vi "Begin.vi"() -> (0 "error out":errorcluster)   [LabVIEW 2012]
doc: "Called before other user functions, this VI is expected to open initial I/O refnums, load in file data, and do all program initialization. Notice that the <B>error out</B> terminal is simply used for data flow. Wiring it to other structures or subVIs ensures that this VI runs first."
uses:
  <vilib>/Rock Robotics/WPI/Joystick/WPI_JoystickDeviceEnum.ctl
  <vilib>/Rock Robotics/SystemInterfaces/Typedef/FPGA_TypedefDigitalModule.ctl
  <vilib>/Rock Robotics/SystemInterfaces/Typedef/FPGA_TypedefSolenoidModule.ctl
  <vilib>/Rock Robotics/WPI/Solenoid/WPI_SolenoidChannel.ctl
  <vilib>/Rock Robotics/WPI/Solenoid/WPI_SolenoidValue.ctl
  <vilib>/Rock Robotics/WPI/Camera/WPI_CameraImageSize.ctl
  <vilib>/Rock Robotics/WPI/Camera/WPI_CameraWhite Balance Values.ctl
  <vilib>/Rock Robotics/WPI/Camera/WPI_CameraExposure Values.ctl
  <vilib>/Rock Robotics/WPI/Camera/WPI_CameraFrameRate.ctl
  <vilib>/Rock Robotics/SystemInterfaces/DIO/FPGA_DIOChannel.ctl
  <vilib>/Rock Robotics/SystemInterfaces/DIO/FPGA_DIORelayChannel.ctl
  <vilib>/Rock Robotics/SystemInterfaces/DIO/FPGA_DIOPWMChannel.ctl
  <vilib>/Rock Robotics/WPI/Solenoid/WPI_SolenoidOpenDouble.vi
  <vilib>/Rock Robotics/WPI/Solenoid/WPI_SolenoidSetEnum.vi
  <vilib>/Rock Robotics/WPI/Compressor/WPI_CompressorGetSetRefNum.vi
  <vilib>/Rock Robotics/WPI/Counter/WPI_CounterDigitalInputToDigitalSource.vi
  <vilib>/Rock Robotics/WPI/MotorControl/WPI_MotorControlOpen Victor.vi
  <vilib>/Rock Robotics/WPI/RobotDrive/WPI_RobotDriveOpen2MotorWithVictor.vi
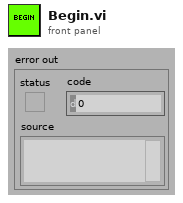
[diagram p1: front panel]
types:
  T1 = typedef "WPI_JoystickDeviceEnum.ctl" = enum16{"USB 1", "USB 2", "USB 3", "USB 4", "Kinect 1", "Kinect 2"}
  T2 = typedef "FPGA_TypedefDigitalModule.ctl" = enum16{"Digital Module 1", "Digital Module 2"}
  T3 = typedef "WPI_CameraFrameRate.ctl" = u32
  T4 = typedef "WPI_CameraExposure Values.ctl" = enum16{"Auto", "Flicker-free 50 Hz", "Flicker-free 60 Hz", "Hold current"}
  T5 = typedef "WPI_CameraWhite Balance Values.ctl" = enum16{"Auto", "Fixed indoor", "Fixed outdoor 1", "Fixed outdoor 2", "Fixed fluorescent 1", "Fixed fluorescent 2", "Hold current"}
  T6 = typedef "WPI_CameraImageSize.ctl" = enum16{"640x480", "320x240", "160x120"}
  T7 = typedef "WPI_CameraDevRef.ctl" = cluster{"Camera Address":string, "CameraStatus":errorcluster, "Acquire Image Notifier":refnum<notifier>}
  T8 = typedef "FPGA_DIOChannel.ctl" = enum8{"DIO 1", "DIO 2", "DIO 3", "DIO 4", "DIO 5", "DIO 6", "DIO 7", "DIO 8", "DIO 9", "DIO 10", "DIO 11", "DIO 12", "DIO 13", "DIO 14", "Invalid"}
  T9 = typedef "FPGA_DIOPWMChannel.ctl" = enum8{"PWM 1", "PWM 2", "PWM 3", "PWM 4", "PWM 5", "PWM 6", "PWM 7", "PWM 8", "PWM 9", "PWM 10", "Invalid"}
  T10 = typedef "WPI_DigitalInputDevRef.ctl" = cluster{"DevStatus":errorcluster, "DIO Channel":T8, "Digital Module":T2}
  T11 = typedef "WPI_RobotDriveDevRef.ctl" = cluster{"DevStatus":errorcluster, "Motors[]":T12[], "Square Inputs":bool, "Max Output":dbl, "Isochronous":bool}
  T12 = typedef "WPI_MotorControlDeviceRef.ctl" = cluster{"DeviceStatus":errorcluster, "Type":enum16{"PWM", "CAN"}, "PWM":cluster{"Digital Module":T2, "PWM Channel":T9, "DeadBand":T13}, "CAN":cluster{"Device Number":u8, "Control Mode":T14, "Semaphore":T15, "Max Vout":dbl}, "Invert":bool, "TransformRef":T16, "InvTransformRef":T16}
  T13 = typedef "WPI_PWMDeadband.ctl" = cluster{"Name":string, "maxPositivePwm":i32, "minPositivePwm":i32, "centerPwm":i32, "maxNegativePwm":i32, "minNegativePwm":i32, "angularRange":u16}
  T14 = typedef "WPI_CANJaguar_ControlMode.ctl" = enum8{"Percent VBus", "Current", "Speed", "Position", "Voltage"}
  T15 = typedef "Semaphore RefNum" = refnum<k1>
  T16 = typedef "WPI_PWMTransform_ConPane.ctl" = refnum<vi>
  T17 = typedef "FPGA_CounterEncoderSourceConvertionLVSourceType.ctl" = cluster{"DevStatus":errorcluster, "AnalogTriggerMode?":bool, "DigitalMode":cluster{"Digital Module":T2, "DIO Channel":T18}, "AnalogTriggerMode":cluster{"AnalogTriggerIndex":T19, "OutputType":T20}}
  T18 = typedef "FPGA_DIODigitalSourceChannel.ctl" = enum8{"DIO 1", "DIO 2", "DIO 3", "DIO 4", "DIO 5", "DIO 6", "DIO 7", "DIO 8", "DIO 9", "DIO 10", "DIO 11", "DIO 12", "DIO 13", "DIO 14", "Disabled"}
  T19 = typedef "FPGA_AnalogTriggerIndex.ctl" = enum8{"Trig 0", "Trig 1", "Trig 2", "Trig 3", "Trig 4", "Trig 5", "Trig 6", "Trig 7", "Invalid"}
  T20 = typedef "FPGA_AnalogTriggerOutType.ctl" = enum16{"InWindow", "TriggerState", "Rising", "Falling"}
  T21 = typedef "WPI_EncoderDevRef.ctl" = cluster{"DevStatus":errorcluster, "EncoderIndex":T22, "CounterIndex":T23, "DistancePerCount":dbl, "Decoding Type":T24}
  T22 = typedef "FPGA_EncoderIdx.ctl" = enum8{"Enc 0", "Enc 1", "Enc 2", "Enc 3", "Invalid"}
  T23 = typedef "FPGA_CounterCtrSystemIndex.ctl" = enum8{"Ctr 0", "Ctr 1", "Ctr 2", "Ctr 3", "Ctr 4", "Ctr 5", "Ctr 6", "Ctr 7", "Invalid"}
  T24 = typedef "WPI_EncoderType.ctl" = enum16{"1x", "2x", "4x"}
  T25 = typedef "WPI_SolenoidValue.ctl" = enum16{"Off", "On", "Forward", "Reverse"}
  T26 = typedef "WPI_SolenoidChannel.ctl" = enum8{"Solenoid 1", "Solenoid 2", "Solenoid 3", "Solenoid 4", "Solenoid 5", "Solenoid 6", "Solenoid 7", "Solenoid 8", "Invalid"}
  T27 = typedef "FPGA_TypedefSolenoidModule.ctl" = enum16{"Solenoid Module 1", "Solenoid Module 2"}
  T28 = typedef "WPI_SolenoidDevRef.ctl" = cluster{"DevStatus":errorcluster, "Solenoid Module":T27, "Forward Solenoid Channel":T26, "Reverse Solenoid Channel":T26}
  T29 = typedef "FPGA_DIORelayChannel.ctl" = enum8{"Relay 1", "Relay 2", "Relay 3", "Relay 4", "Relay 5", "Relay 6", "Relay 7", "Relay 8", "Invalid"}
  T30 = typedef "WPI_CompressorDevRef.ctl" = cluster{"DevStatus":errorcluster, "DigitalInputDevRef":T10, "RelayDevRef":T31}
  T31 = typedef "WPI_RelayDevRef.ctl" = cluster{"DevStatus":errorcluster, "Relay Channel":T29, "Digital Module":T2, "Relay Direction":T32}
  T32 = typedef "WPI_RelayDirection.ctl" = enum16{"Both directions", "Forward only", "Reverse only"}
  T33 = typedef "WPI_JoystickDevRef.ctl" = cluster{"Device":T1}
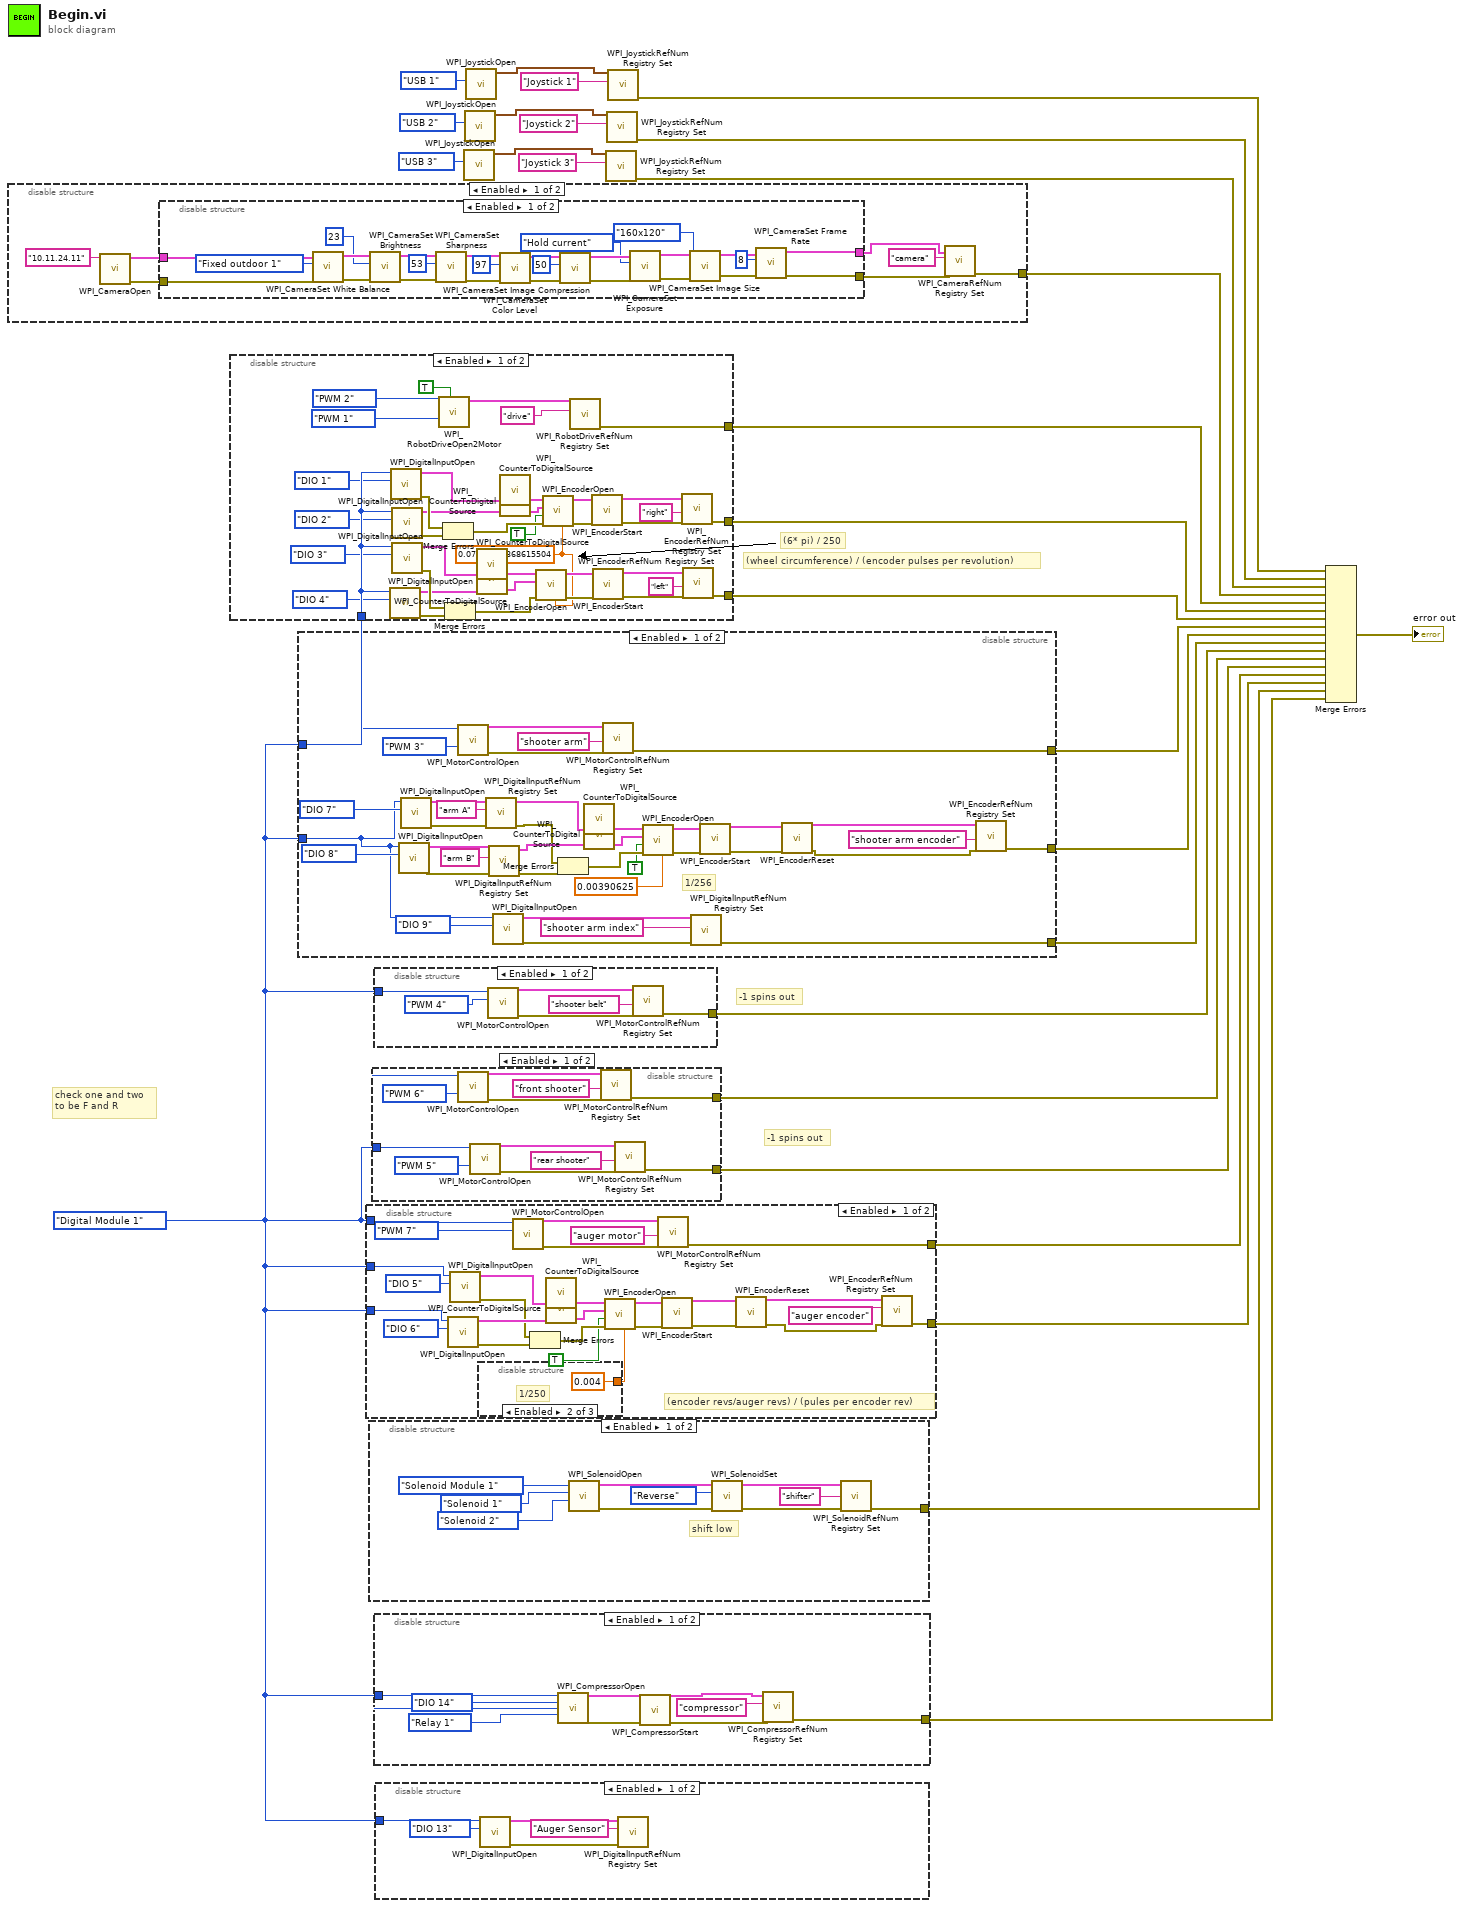
[diagram p0: block diagram]
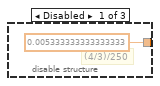
[diagram p4: hidden frame]
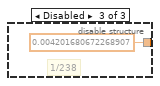
[diagram p5: hidden frame]
diagram:
  w1 = FPGA_TypedefDigitalModule."Digital Module 1" ("Digital Module (Module 1)")
  # "-1 spins out"
  # "-1 spins out"
  # "(wheel circumference) / (encoder pulses per revolution)"
  # "(6* pi) / 250"
  # "check one and two\nto be F and R"
  n1 = disable-structure shown="Enabled" {
    disable-tunnel: [w29 _] -> w16
    frame Enabled {
      n2 = call <vilib>:"WPI_CameraOpen.vi"("Camera Address"="10.11.24.11") -> ("error out"=w31:errorcluster, "CameraDevRef"=w33:T7)  [unwired: 9 in]
      n3 = disable-structure shown="Enabled" {
        disable-tunnel: w33 -> [w59 w63]
        disable-tunnel: [w37 w63] -> w32
        disable-tunnel: w31 -> [w46 w62]
        disable-tunnel: [w36 w62] -> w30
        frame Enabled {
          n4 = call <vilib>:"WPI_CameraSet White Balance.vi"("error in (no error)"=w46, "White Balance"=WPI_CameraWhite_Balance_Values."Fixed outdoor 1", "CameraDevRef"=w59) -> ("error out"=w47:errorcluster, "CameraDevRef Out"=w58:T7)  [unwired: 7 in]
          n5 = call <vilib>:"WPI_CameraSet Brightness.vi"("error in (no error)"=w47, "Brightness"=23, "CameraDevRef"=w58) -> ("error out"=w48:errorcluster, "CameraDevRef Out"=w57:T7)  [unwired: 7 in]
          n6 = call <vilib>:"WPI_CameraSet Sharpness.vi"("error in (no error)"=w48, "Sharpness"=53, "CameraDevRef"=w57) -> ("error out"=w49:errorcluster, "CameraDevRef Out"=w56:T7)  [unwired: 7 in]
          n7 = call <vilib>:"WPI_CameraSet Color Level.vi"("error in (no error)"=w49, "Color Level"=97, "CameraDevRef"=w56) -> ("error out"=w50:errorcluster, "CameraDevRef Out"=w55:T7)  [unwired: 7 in]
          n8 = call <vilib>:"WPI_CameraSet Image Compression.vi"("error in (no error)"=w50, "Compression"=50, "CameraDevRef"=w55) -> ("error out"=w61:errorcluster, "CameraDevRef Out"=w60:T7)  [unwired: 7 in]
          n9 = call <vilib>:"WPI_CameraSet Exposure.vi"("error in (no error)"=w61, "Exposure"=WPI_CameraExposure_Values."Hold current", "CameraDevRef"=w60) -> ("error out"=w51:errorcluster, "CameraDevRef Out"=w54:T7)  [unwired: 7 in]
          n10 = call <vilib>:"WPI_CameraSet Image Size.vi"("error in (no error)"=w51, "Image Size"=WPI_CameraImageSize."160x120", "CameraDevRef"=w54) -> ("error out"=w52:errorcluster, "CameraDevRef Out"=w53:T7)  [unwired: 7 in]
          n11 = call <vilib>:"WPI_CameraSet Frame Rate.vi"("error in (no error)"=w52, "Frame Rate (fps)"=T3 8, "CameraDevRef"=w53) -> ("error out"=w36:errorcluster, "CameraDevRef Out"=w37:T7)  [unwired: 7 in]
        }
        frame Disabled {
        }
      }
      n12 = call <vilib>:"WPI_CameraRefNum Registry Set.vi"("error in (no error)"=w30, "refnum name"="camera", "CameraDevRef"=w32) -> ("error out"=w29:errorcluster)  [unwired: 7 in, 1 out]
    }
    frame Disabled {
    }
  }
  n13 = disable-structure shown="Enabled" {
    disable-tunnel: w1 -> [w82 _]
    disable-tunnel: [w76 _] -> w15
    disable-tunnel: [w75 _] -> w14
    disable-tunnel: [w74 _] -> w13
    frame Enabled {
      w77 = 0.07539822368615504 ("DistancePerCount")
      n14 = call <vilib>:"WPI_DigitalInputOpen.vi"("DIO Channel"=FPGA_DIOChannel."DIO 4", "Digital Module (Module 1)"=w82) -> ("error out"=w73:errorcluster, "DigitalInputDevRef"=w66:T10)  [unwired: 8 in]
      n15 = call <vilib>:"WPI_DigitalInputOpen.vi"("DIO Channel"=FPGA_DIOChannel."DIO 1", "Digital Module (Module 1)"=w82) -> ("error out"=w68:errorcluster, "DigitalInputDevRef"=w86:T10)  [unwired: 8 in]
      n16 = call <vilib>:"WPI_DigitalInputOpen.vi"("DIO Channel"=FPGA_DIOChannel."DIO 2", "Digital Module (Module 1)"=w82) -> ("error out"=w70:errorcluster, "DigitalInputDevRef"=w67:T10)  [unwired: 8 in]
      n17 = call <vilib>:"WPI_DigitalInputOpen.vi"("DIO Channel"=FPGA_DIOChannel."DIO 3", "Digital Module (Module 1)"=w82) -> ("error out"=w71:errorcluster, "DigitalInputDevRef"=w100:T10)  [unwired: 8 in]
      n18 = call-poly <vilib>:"WPI_RobotDriveOpen2Motor.vi"("Left Motor Inverted"=TRUE, "Right Motor"=FPGA_DIOPWMChannel."PWM 1", "Left Motor"=FPGA_DIOPWMChannel."PWM 2") -> ("RobotDriveDevRef"=w102:T11)  [unwired: 7 in, 1 out]
      n19 = Merge Errors(w68, w70) -> (w69:errorcluster)
      n20 = Merge Errors(w71, w73) -> (w72:errorcluster)
      n21 = call-poly <vilib>:"WPI_CounterToDigitalSource.vi"("DigitalInputDevRef"=w100) -> ("Digital Source"=w93:T17)  [unwired: 6 in]
      n22 = call-poly <vilib>:"WPI_CounterToDigitalSource.vi"("DigitalInputDevRef"=w66) -> ("Digital Source"=w94:T17)  [unwired: 6 in]
      n23 = call-poly <vilib>:"WPI_CounterToDigitalSource.vi"("DigitalInputDevRef"=w86) -> ("Digital Source"=w92:T17)  [unwired: 6 in]
      n24 = call-poly <vilib>:"WPI_CounterToDigitalSource.vi"("DigitalInputDevRef"=w67) -> ("Digital Source"=w91:T17)  [unwired: 6 in]
      n25 = call <vilib>:"WPI_EncoderOpen.vi"("DistancePerCount"=w77, "error in (no error)"=w72, "BSource"=w94, "ASource"=w93) -> ("error out"=w95:errorcluster, "EncoderDevRef"=w96:T21)  [unwired: 6 in]
      n26 = call <vilib>:"WPI_EncoderOpen.vi"("DistancePerCount"=w77, "error in (no error)"=w69, "Invert Direction (False)"=TRUE, "BSource"=w91, "ASource"=w92) -> ("error out"=w90:errorcluster, "EncoderDevRef"=w89:T21)  [unwired: 5 in]
      n27 = call <vilib>:"WPI_RobotDriveRefNum Registry Set.vi"("refnum name"="drive", "RobotDriveDevRef"=w102) -> ("error out"=w76:errorcluster)  [unwired: 8 in, 1 out]
      n28 = call <vilib>:"WPI_EncoderStart.vi"("error in (no error)"=w90, "EncoderDevRef"=w89) -> ("error out"=w88:errorcluster, "EncoderDevRef"=w87:T21)  [unwired: 8 in]
      n29 = call <vilib>:"WPI_EncoderStart.vi"("error in (no error)"=w95, "EncoderDevRef"=w96) -> ("error out"=w97:errorcluster, "EncoderDevRef"=w98:T21)  [unwired: 8 in]
      n30 = call <vilib>:"WPI_EncoderRefNum Registry Set.vi"("error in (no error)"=w88, "refnum name"="right", "EncoderDevRef"=w87) -> ("error out"=w75:errorcluster)  [unwired: 7 in, 1 out]
      n31 = call <vilib>:"WPI_EncoderRefNum Registry Set.vi"("error in (no error)"=w97, "refnum name"="left", "EncoderDevRef"=w98) -> ("error out"=w74:errorcluster)  [unwired: 7 in, 1 out]
    }
    frame Disabled {
    }
  }
  n32 = disable-structure shown="Enabled" {
    disable-tunnel: w1 -> [w135 _]
    disable-tunnel: w1 -> [w125 _]
    disable-tunnel: [w121 _] -> w12
    disable-tunnel: [w120 _] -> w11
    disable-tunnel: [w119 _] -> w10
    frame Enabled {
      # "1/256"
      n33 = call <vilib>:"WPI_DigitalInputOpen.vi"("DIO Channel"=FPGA_DIOChannel."DIO 8", "Digital Module (Module 1)"=w125) -> ("error out"=w108:errorcluster, "DigitalInputDevRef"=w109:T10)  [unwired: 8 in]
      n34 = call <vilib>:"WPI_DigitalInputOpen.vi"("DIO Channel"=FPGA_DIOChannel."DIO 7", "Digital Module (Module 1)"=w125) -> ("error out"=w111:errorcluster, "DigitalInputDevRef"=w112:T10)  [unwired: 8 in]
      n35 = call-poly <vilib>:"WPI_MotorControlOpen.vi"("PWM Channel"=FPGA_DIOPWMChannel."PWM 3", "Digital Module (Module 1)"=w135) -> ("error out"=w137:errorcluster, "MotorControlDeviceRef"=w138:T12)  [unwired: 8 in]
      n36 = call <vilib>:"WPI_DigitalInputRefNum Registry Set.vi"("error in (no error)"=w111, "refnum name"="arm A", "DigitalInputDevRef"=w112) -> ("error out"=w104:errorcluster, "DigitalInputDevRef"=w106:T10)  [unwired: 7 in]
      n37 = call <vilib>:"WPI_DigitalInputRefNum Registry Set.vi"("error in (no error)"=w108, "refnum name"="arm B", "DigitalInputDevRef"=w109) -> ("error out"=w103:errorcluster, "DigitalInputDevRef"=w105:T10)  [unwired: 7 in]
      n38 = call <vilib>:"WPI_DigitalInputOpen.vi"("DIO Channel"=FPGA_DIOChannel."DIO 9", "Digital Module (Module 1)"=w125) -> ("error out"=w123:errorcluster, "DigitalInputDevRef"=w124:T10)  [unwired: 8 in]
      n39 = Merge Errors(w104, w103) -> (w118:errorcluster)
      n40 = call-poly <vilib>:"WPI_CounterToDigitalSource.vi"("DigitalInputDevRef"=w106) -> ("Digital Source"=w133:T17)  [unwired: 6 in]
      n41 = call-poly <vilib>:"WPI_CounterToDigitalSource.vi"("DigitalInputDevRef"=w105) -> ("Digital Source"=w132:T17)  [unwired: 6 in]
      n42 = call <vilib>:"WPI_MotorControlRefNum Registry Set.vi"("error in (no error)"=w137, "refnum name"="shooter arm", "MotorControlDevRef"=w138) -> ("error out"=w121:errorcluster)  [unwired: 7 in, 1 out]
      n43 = call <vilib>:"WPI_EncoderOpen.vi"("DistancePerCount"=0.00390625, "error in (no error)"=w118, "Invert Direction (False)"=TRUE, "BSource"=w132, "ASource"=w133) -> ("error out"=w131:errorcluster, "EncoderDevRef"=w130:T21)  [unwired: 5 in]
      n44 = call <vilib>:"WPI_DigitalInputRefNum Registry Set.vi"("error in (no error)"=w123, "refnum name"="shooter arm index", "DigitalInputDevRef"=w124) -> ("error out"=w119:errorcluster)  [unwired: 7 in, 1 out]
      n45 = call <vilib>:"WPI_EncoderStart.vi"("error in (no error)"=w131, "EncoderDevRef"=w130) -> ("error out"=w115:errorcluster, "EncoderDevRef"=w116:T21)  [unwired: 8 in]
      n46 = call <vilib>:"WPI_EncoderReset.vi"("error in (no error)"=w115, "EncoderDevRef"=w116) -> ("error out"=w114:errorcluster, "EncoderDevRef"=w113:T21)  [unwired: 8 in]
      n47 = call <vilib>:"WPI_EncoderRefNum Registry Set.vi"("error in (no error)"=w114, "refnum name"="shooter arm encoder", "EncoderDevRef"=w113) -> ("error out"=w120:errorcluster)  [unwired: 7 in, 1 out]
    }
    frame Disabled {
    }
  }
  n48 = disable-structure shown="Enabled" {
    disable-tunnel: w1 -> [w152 _]
    disable-tunnel: w1 -> [w151 _]
    disable-tunnel: w1 -> [w150 _]
    disable-tunnel: [w149 _] -> w6
    disable-tunnel: [w148 _] -> w5
    frame Enabled {
      # "(encoder revs/auger revs) / (pules per encoder rev)"
      n49 = call <vilib>:"WPI_DigitalInputOpen.vi"("DIO Channel"=FPGA_DIOChannel."DIO 6", "Digital Module (Module 1)"=w150) -> ("error out"=w147:errorcluster, "DigitalInputDevRef"=w155:T10)  [unwired: 8 in]
      n50 = call <vilib>:"WPI_DigitalInputOpen.vi"("DIO Channel"=FPGA_DIOChannel."DIO 5", "Digital Module (Module 1)"=w151) -> ("error out"=w145:errorcluster, "DigitalInputDevRef"=w158:T10)  [unwired: 8 in]
      n51 = disable-structure shown="Enabled" {
        disable-tunnel: [0.005333333333333333 ("DistancePerCount") 0.004 ("DistancePerCount") 0.004201680672268907 ("DistancePerCount")] -> w154
        frame Disabled {
          # "(4/3)/250"
        }
        frame Enabled {
          # "1/250"
        }
        frame Disabled {
          # "1/238"
        }
      }
      n52 = call-poly <vilib>:"WPI_MotorControlOpen.vi"("PWM Channel"=FPGA_DIOPWMChannel."PWM 7", "Digital Module (Module 1)"=w152) -> ("error out"=w165:errorcluster, "MotorControlDeviceRef"=w166:T12)  [unwired: 8 in]
      n53 = Merge Errors(w145, w147) -> (w146:errorcluster)
      n54 = call-poly <vilib>:"WPI_CounterToDigitalSource.vi"("DigitalInputDevRef"=w158) -> ("Digital Source"=w163:T17)  [unwired: 6 in]
      n55 = call-poly <vilib>:"WPI_CounterToDigitalSource.vi"("DigitalInputDevRef"=w155) -> ("Digital Source"=w162:T17)  [unwired: 6 in]
      n56 = call <vilib>:"WPI_EncoderOpen.vi"("DistancePerCount"=w154, "error in (no error)"=w146, "Invert Direction (False)"=TRUE, "BSource"=w162, "ASource"=w163) -> ("error out"=w161:errorcluster, "EncoderDevRef"=w160:T21)  [unwired: 5 in]
      n57 = call <vilib>:"WPI_MotorControlRefNum Registry Set.vi"("error in (no error)"=w165, "refnum name"="auger motor", "MotorControlDevRef"=w166) -> ("error out"=w149:errorcluster)  [unwired: 7 in, 1 out]
      n58 = call <vilib>:"WPI_EncoderStart.vi"("error in (no error)"=w161, "EncoderDevRef"=w160) -> ("error out"=w142:errorcluster, "EncoderDevRef"=w143:T21)  [unwired: 8 in]
      n59 = call <vilib>:"WPI_EncoderReset.vi"("error in (no error)"=w142, "EncoderDevRef"=w143) -> ("error out"=w141:errorcluster, "EncoderDevRef"=w140:T21)  [unwired: 8 in]
      n60 = call <vilib>:"WPI_EncoderRefNum Registry Set.vi"("error in (no error)"=w141, "refnum name"="auger encoder", "EncoderDevRef"=w140) -> ("error out"=w148:errorcluster)  [unwired: 7 in, 1 out]
    }
    frame Disabled {
    }
  }
  n61 = disable-structure shown="Enabled" {
    disable-tunnel: [w175 _] -> w4
    frame Enabled {
      # "shift low"
      n62 = call-poly <vilib>:"WPI_SolenoidOpen.vi"("Reverse Solenoid Channel"=WPI_SolenoidChannel."Solenoid 2", "Forward Solenoid Channel"=WPI_SolenoidChannel."Solenoid 1", "Solenoid Module (Module 1)"=FPGA_TypedefSolenoidModule."Solenoid Module 1") -> ("error out"=w172:errorcluster, "SolenoidDevRef"=w173:T28)  [unwired: 7 in]
      n63 = call-poly <vilib>:"WPI_SolenoidSet.vi"("error in (no error)"=w172, "Value"=WPI_SolenoidValue."Reverse", "SolenoidDevRef"=w173) -> ("error out"=w171:errorcluster, "SolenoidDevRef"=w170:T28)  [unwired: 7 in]
      n64 = call <vilib>:"WPI_SolenoidRefNum Registry Set.vi"("error in (no error)"=w171, "refnum name"="shifter", "SolenoidDevRef"=w170) -> ("error out"=w175:errorcluster)  [unwired: 7 in, 1 out]
    }
    frame Disabled {
    }
  }
  n65 = disable-structure shown="Enabled" {
    disable-tunnel: w1 -> [w186 _]
    disable-tunnel: [w181 _] -> w8
    disable-tunnel: [w180 _] -> w7
    frame Enabled {
      n66 = call-poly <vilib>:"WPI_MotorControlOpen.vi"("PWM Channel"=FPGA_DIOPWMChannel."PWM 6", "Digital Module (Module 1)"=w186) -> ("error out"=w184:errorcluster, "MotorControlDeviceRef"=w183:T12)  [unwired: 8 in]
      n67 = call-poly <vilib>:"WPI_MotorControlOpen.vi"("PWM Channel"=FPGA_DIOPWMChannel."PWM 5", "Digital Module (Module 1)"=w186) -> ("error out"=w188:errorcluster, "MotorControlDeviceRef"=w189:T12)  [unwired: 8 in]
      n68 = call <vilib>:"WPI_MotorControlRefNum Registry Set.vi"("error in (no error)"=w184, "refnum name"="front shooter", "MotorControlDevRef"=w183) -> ("error out"=w181:errorcluster)  [unwired: 7 in, 1 out]
      n69 = call <vilib>:"WPI_MotorControlRefNum Registry Set.vi"("error in (no error)"=w188, "refnum name"="rear shooter", "MotorControlDevRef"=w189) -> ("error out"=w180:errorcluster)  [unwired: 7 in, 1 out]
    }
    frame Disabled {
    }
  }
  n70 = disable-structure shown="Enabled" {
    disable-tunnel: w1 -> [w192 _]
    disable-tunnel: [w191 _] -> w9
    frame Enabled {
      n71 = call-poly <vilib>:"WPI_MotorControlOpen.vi"("PWM Channel"=FPGA_DIOPWMChannel."PWM 4", "Digital Module (Module 1)"=w192) -> ("error out"=w195:errorcluster, "MotorControlDeviceRef"=w194:T12)  [unwired: 8 in]
      n72 = call <vilib>:"WPI_MotorControlRefNum Registry Set.vi"("error in (no error)"=w195, "refnum name"="shooter belt", "MotorControlDevRef"=w194) -> ("error out"=w191:errorcluster)  [unwired: 7 in, 1 out]
    }
    frame Disabled {
    }
  }
  n73 = disable-structure shown="Enabled" {
    disable-tunnel: w1 -> [w204 _]
    disable-tunnel: [w201 _] -> w3
    frame Enabled {
      n74 = call <vilib>:"WPI_CompressorOpen.vi"("Pressure Switch Digital Module (Module 1)"=w204, "Pressure Switch DIO Channel"=FPGA_DIOChannel."DIO 14", "Relay Digital Module (Module 1)"=w204, "Relay Channel"=FPGA_DIORelayChannel."Relay 1") -> ("CompressorDevRef"=w200:T30, "error out"=w199:errorcluster)  [unwired: 10 in]
      n75 = call <vilib>:"WPI_CompressorStart.vi"("error in (no error)"=w199, "CompressorDevRef"=w200) -> ("error out"=w198:errorcluster, "CompressorDevRef"=w197:T30)  [unwired: 8 in]
      n76 = call <vilib>:"WPI_CompressorRefNum Registry Set.vi"("error in (no error)"=w198, "refnum name"="compressor", "CompressorDevRef"=w197) -> ("error out"=w201:errorcluster)  [unwired: 7 in, 1 out]
    }
    frame Disabled {
    }
  }
  n77 = disable-structure shown="Enabled" {
    disable-tunnel: w1 -> [w210 _]
    frame Enabled {
      n78 = call <vilib>:"WPI_DigitalInputOpen.vi"("DIO Channel"=FPGA_DIOChannel."DIO 13", "Digital Module (Module 1)"=w210) -> ("error out"=w208:errorcluster, "DigitalInputDevRef"=w207:T10)  [unwired: 8 in]
      n79 = call <vilib>:"WPI_DigitalInputRefNum Registry Set.vi"("error in (no error)"=w208, "refnum name"="Auger Sensor", "DigitalInputDevRef"=w207) -> ()  [unwired: 7 in, 2 out]
    }
    frame Disabled {
    }
  }
  n80 = call <vilib>:"WPI_JoystickOpen.vi"("JoystickDevice"=WPI_JoystickDeviceEnum."USB 3") -> ("JoystickDevRef"=w27:T33)  [unwired: 10 in]
  n81 = call <vilib>:"WPI_JoystickOpen.vi"("JoystickDevice"=WPI_JoystickDeviceEnum."USB 2") -> ("JoystickDevRef"=w24:T33)  [unwired: 10 in]
  n82 = call <vilib>:"WPI_JoystickOpen.vi"("JoystickDevice"=WPI_JoystickDeviceEnum."USB 1") -> ("JoystickDevRef"=w21:T33)  [unwired: 10 in]
  n83 = call <vilib>:"WPI_JoystickRefNum Registry Set.vi"("refnum name"="Joystick 3", "JoystickDevRef"=w27) -> ("error out"=w17:errorcluster)  [unwired: 8 in, 1 out]
  n84 = call <vilib>:"WPI_JoystickRefNum Registry Set.vi"("refnum name"="Joystick 2", "JoystickDevRef"=w24) -> ("error out"=w18:errorcluster)  [unwired: 8 in, 1 out]
  n85 = call <vilib>:"WPI_JoystickRefNum Registry Set.vi"("refnum name"="Joystick 1", "JoystickDevRef"=w21) -> ("error out"=w19:errorcluster)  [unwired: 8 in, 1 out]
  n86 = Merge Errors(w19, w18, w17, w16, w15, w14, w13, w12, w11, w10, w9, w8, w7, w6, w5, w4, w3) -> (→"error out":errorcluster)
